vi "AssertValueByArrayPath.vi"(0 "VI Reference In":refnum<vi>, 1 "Test Label":string, 2 "delimiter (>>)":string=">>", 3 "Assert Only? (F)":bool, 5 "Control Path":string, 7 "Focus Item Path":string[](array[string]), 11 "Error In":errorcluster, 12 "Assert Interval(10 ms)":u32=10, 13 "Timeout(5 sec)":dbl=5.0) -> (4 "VI Reference Out":refnum<vi>, 6 "Asserted Value":string[](array[string]), 15 "Error Out":errorcluster)   [LabVIEW 2016, in "Drona.lvlib" / "AssertControlValue.lvlib" / "AssertTree.lvlib"]
doc: "Asserts if the focus item names given as a array of hierarchical path for multi-select tree controls are equal.\n\nHierarchical path represent their corresponding parents of an item from its origin. Use the delimiters '>>' between each hierarchy in the path.\n\nFor example to select the item 'Child3', give the hierarchical path as \"<b>Parent1</b>(top level parent in tree)<b>>>Child1</b>(children for parent1)<b>>>Child2</b>(children for child1)<b>>>Child3</b>(children for child2)\"\n\nThe input control name is given as a string , incase of path, use delimiters inbetween the path.\nThis VI gets the value of the control, untill the value is equal to the input value."
uses:
  AssertTree.lvlib
  Get/GetControlRef/GetControlRefByPath.vi
  <vilib>/Utility/error.llb/Error Cluster From Error Code.vi
  <vilib>/addons/_JKI Toolkits/Caraya/classes/Assert/Assert Equal Value_Variant.vi
  <vilib>/ErrorRing/Error Ring.xnode
  Get/GetControlRef/GetControlRef.lvlib
  <vilib>/addons/_JKI Toolkits/Caraya/classes/Assert/Assert.lvclass
  Drona.lvlib
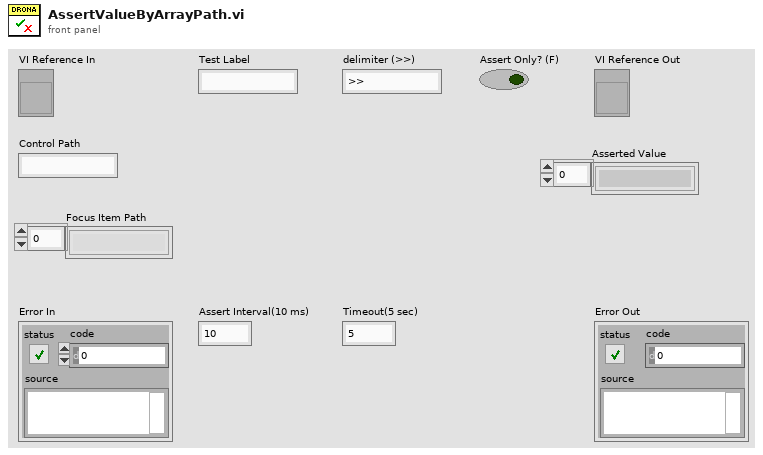
[diagram p1: front panel]
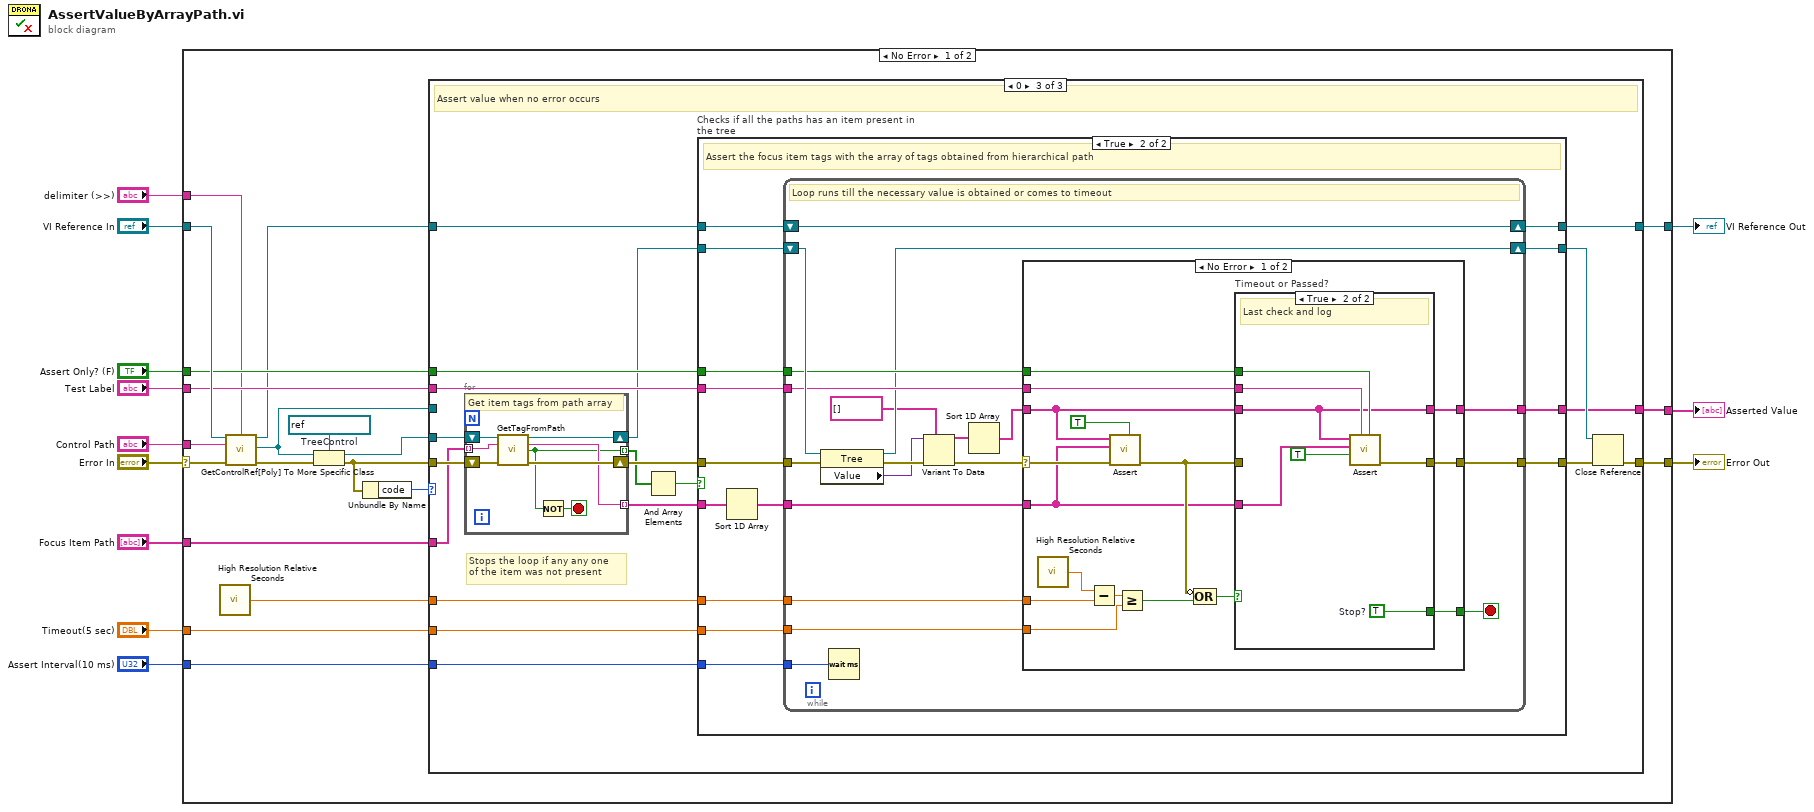
[diagram p0: block diagram]
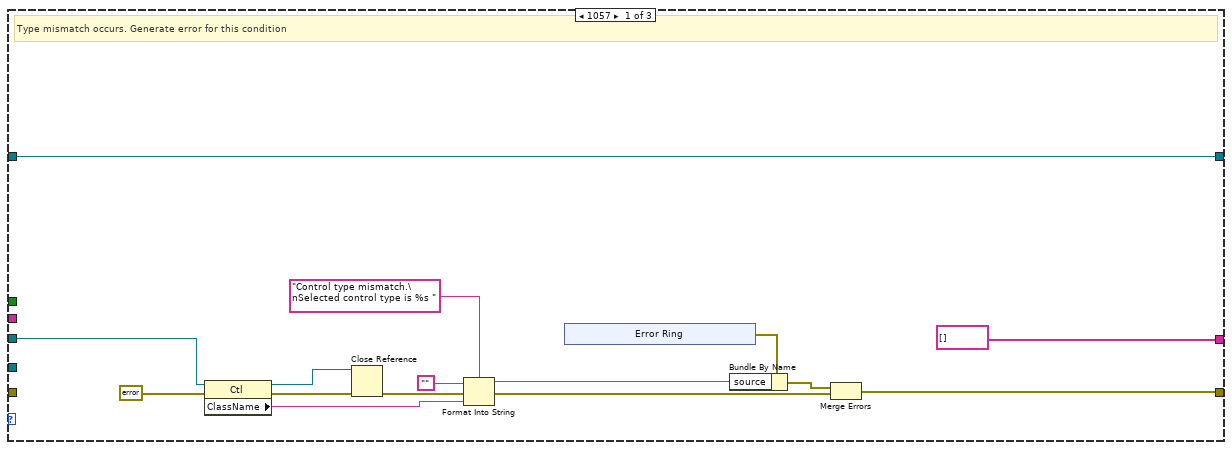
[diagram p2: hidden frame]
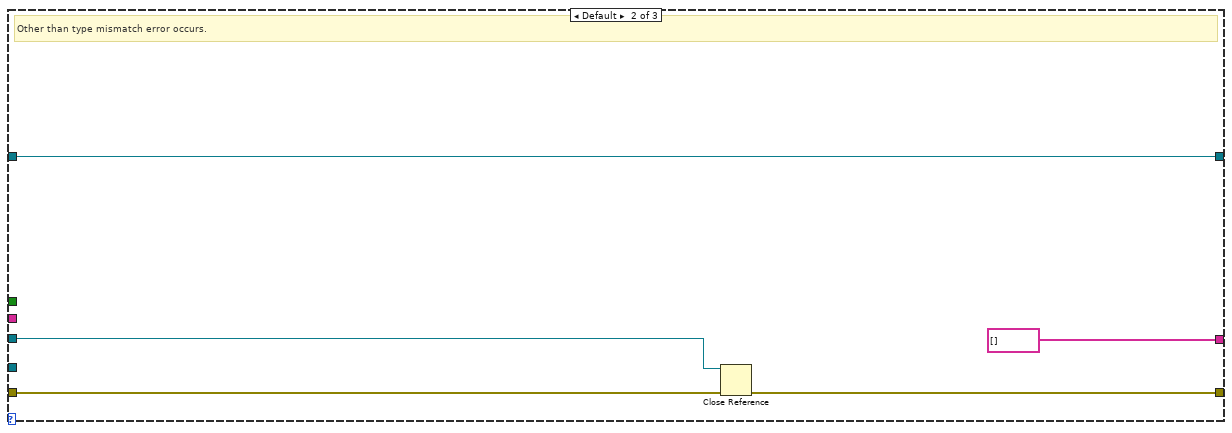
[diagram p3: hidden frame]
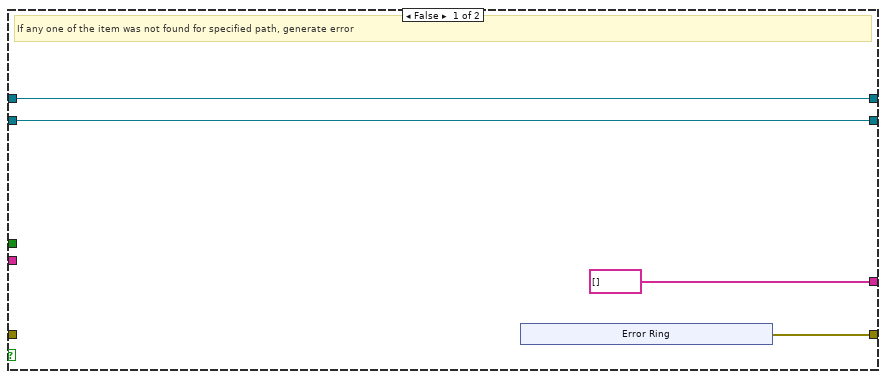
[diagram p4: hidden frame]
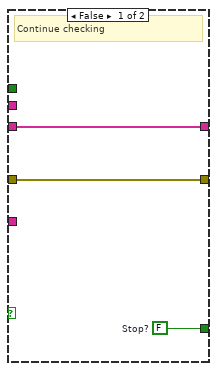
[diagram p5: hidden frame]
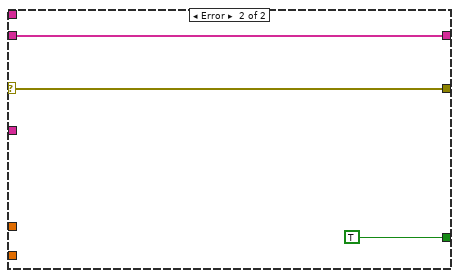
[diagram p6: hidden frame]
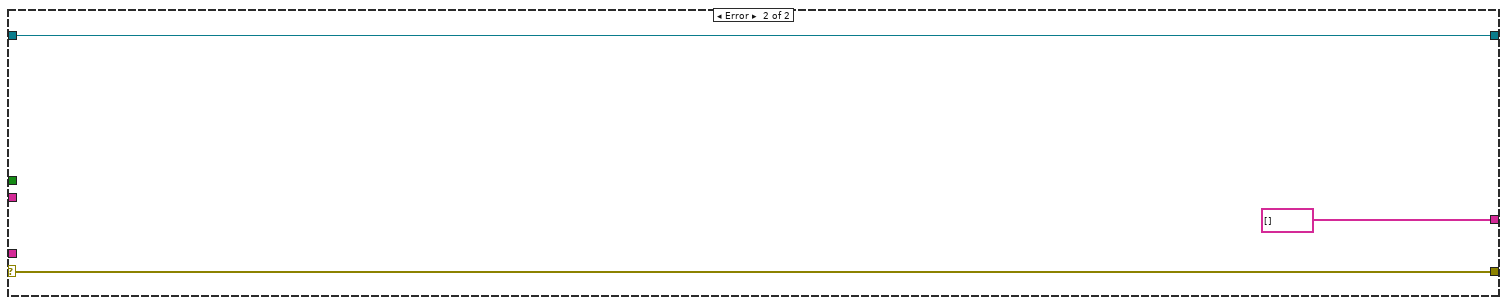
[diagram p7: hidden frame]
diagram:
  n1 = case shown="No Error" "Error In" {
    selector: "Error In" -> [w32 w158]
    tunnel: "Timeout(5 sec)" -> [w19 _]
    tunnel: [w17 w157] -> w11
    tunnel: "Focus Item Path" -> [w21 _]
    tunnel: [w15 w158] -> w10
    tunnel: "Assert Interval(10 ms)" -> [w18 _]
    tunnel: "Test Label" -> [w25 _]
    tunnel: "VI Reference In" -> [w31 w157]
    tunnel: "Control Path" -> [w13 _]
    tunnel: "delimiter (>>)" -> [w14 _]
    tunnel: "Assert Only? (F)" -> [w24 _]
    tunnel: [w16 string[] []] -> w1
    frame No Error {
      w29 = refnum<vi> refnum  # TreeControl
      n2 = call <vilib>:"High Resolution Relative Seconds.vi"() -> ("relative seconds"=w20:dbl)
      n3 = call-poly "GetControlRef[Poly].vi"("VI Reference In"=w31, "delimiter (>>)"=w14, "Control Path"=w13, "error In"=w32) -> ("VI Reference Out"=w23:refnum<vi>, "Ctl Refnum"=w26:refnum<vi>, "error out"=w30:errorcluster)  [unwired: 9 in]
      n4 = To More Specific Class(target class=w29, reference=w26, error in=w30) -> (specific class reference=w27:refnum<vi>, error out=w28:errorcluster)
      n5 = Unbundle By Name(w28) -> ("code"=w22:i32)
      n6 = case shown="0" w22 {
        tunnel: w19 -> [_ _ w76]
        tunnel: [w47 w57 w75] -> w17
        tunnel: w21 -> [_ _ w60]
        tunnel: w18 -> [_ _ w73]
        tunnel: w25 -> [_ _ w72]
        tunnel: w20 -> [_ _ w71]
        tunnel: w23 -> [w47 w57 w70]
        tunnel: [w35 w55 w69] -> w15
        tunnel: w24 -> [_ _ w67]
        tunnel: [string[] [] string[] [] w66] -> w16
        tunnel: w28 -> [_ w56 w65]
        tunnel: w27 -> [_ _ w64]
        tunnel: w26 -> [w34 w54 _]
        frame 1057 {
          # "Type mismatch occurs. Generate error for this condition"
          n7 = property class="Ctl"(reference=w34, error in=errorcluster {"status"=FALSE, "code"=0, "source"=""} ("error out")) -> (reference out=w36:refnum<vi>, error out=w46:errorcluster, "ClassName"=w43:string)
          n8 = Close Reference(reference=w36, error in (no error)=w46) -> (error out=w37:errorcluster)
          n9 = Format Into String(format string="Control type mismatch.\nSelected control type is %s ", initial string="", error in=w37, w43) -> (resulting string=w40:string, error out=w38:errorcluster)
          n10 = xnode "Error Ring"() -> ("error out"=w41:errorcluster)
          n11 = Bundle By Name(cluster=w41, "source"=w40) -> (w39:errorcluster)
          n12 = Merge Errors(w39, w38) -> (w35:errorcluster)
        }
        frame Default {
          # "Other than type mismatch error occurs."
          n13 = Close Reference(reference=w54, error in (no error)=w56) -> (error out=w55:errorcluster)
        }
        frame 0 {
          # "Stops the loop if any any one \nof the item was not present"
          # "Assert value when no error occurs"
          n14 = for {
            tunnel: [w78] -> w63 mode=indexing
            tunnel: [w77] -> w58 mode=indexing
            shift-right: [w82] -> w62
            shift-left: w65 -> [w83]
            shift-right: [w79] -> w61
            shift-left: w64 -> [w81]
            tunnel: w60 -> [w80] mode=indexing
            stop <- w84 stop-if-true
            # "Get item tags from path array"
            n15 = call "GetTagFromPath.vi"("Tree Ref In"=w81, "Hierarchical Path"=w80, "Error In"=w83) -> ("Tree Ref Out"=w79:refnum<vi>, "Item Tag"=w78:string, "Item Found?"=w77:bool, "Error Out"=w82:errorcluster)  [unwired: 9 in]
            n16 = Not(x=w77) -> (.not. x?=w84:bool)
          }
          n17 = And Array Elements(Boolean array=w58) -> (logical AND=w59:bool)
          n18 = case "Checks if all the paths has an item present in the tree" shown="True" w59 {
            tunnel: w76 -> [_ w107]
            tunnel: [w88 w106] -> w75
            tunnel: [w86 w105] -> w74
            tunnel: w73 -> [_ w104]
            tunnel: w72 -> [_ w103]
            tunnel: w71 -> [_ w102]
            tunnel: w70 -> [w88 w101]
            tunnel: [w87 w100] -> w68
            tunnel: w67 -> [_ w99]
            tunnel: [string[] [] w98] -> w66
            tunnel: w63 -> [_ w95]
            tunnel: w61 -> [w87 w96]
            tunnel: w62 -> [_ w97]
            frame False {
              # "If any one of the item was not found for specified path, generate error"
              n19 = xnode "Error Ring"() -> ("error out"=w86:errorcluster)
            }
            frame True {
              # "Assert the focus item tags with the array of tags obtained from hierarchical path"
              n20 = Sort 1D Array(array=w95) -> (sorted array=w94:string[])
              n21 = while {
                tunnel: w94 -> [w114]
                tunnel: w107 -> [w125]
                tunnel: w102 -> [w126]
                tunnel: w97 -> [w120]
                tunnel: [w123] -> w105
                tunnel: w104 -> [w121]
                tunnel: w103 -> [w117]
                shift-right: [w118] -> w106
                shift-left: w101 -> [w118]
                shift-right: [w111] -> w100
                shift-left: w96 -> [w119]
                tunnel: w99 -> [w116]
                tunnel: [w115] -> w98
                stop <- w124 stop-if-true
                # "Loop runs till the necessary value is obtained or comes to timeout"
                n22 = property on="Property Node" class="Tree"(reference=w119, error in=w120) -> (reference out=w111:refnum<vi>, error out=w122:errorcluster, "Value"=w112:variant)
                n23 = Wait (ms)(milliseconds to wait=w121) -> ()  [unwired: 1 out]
                n24 = Variant To Data(error in=w122, type=string[] [], Variant=w112) -> (data=w109:string[], error out=w113:errorcluster)
                n25 = Sort 1D Array(array=w109) -> (sorted array=w108:string[])
                n26 = case shown="No Error" w113 {
                  selector: w113 -> [w138 w155]
                  tunnel: w126 -> [w142 _]
                  tunnel: w125 -> [w139 _]
                  tunnel: [w129 TRUE] -> w124
                  tunnel: [w130 w155] -> w123
                  tunnel: w114 -> [w131 _]
                  tunnel: w108 -> [w132 w153]
                  tunnel: w117 -> [w137 _]
                  tunnel: w116 -> [w128 _]
                  tunnel: [w127 w153] -> w115
                  frame No Error {
                    n27 = call <vilib>:"High Resolution Relative Seconds.vi"() -> ("relative seconds"=w141:dbl)
                    n28 = Subtract(x=w141, y=w142) -> (x-y=w140:dbl)
                    n29 = call-poly <vilib>:"Assert.vi"("Assert Only? (F)"=TRUE, "error in (no error)"=w138, "Y"=w131, "X"=w132) -> ("error out"=w135:errorcluster)  [unwired: 6 in, 1 out]
                    n30 = Greater Or Equal?(x=w140, y=w139) -> (x >= y?=w136:bool)
                    n31 = Compound Arithmetic op=OR(invert w135, w136) -> (w134:bool)
                    n32 = case "Timeout or Passed?" shown="True" w134 {
                      tunnel: w135 -> [w145 _]
                      tunnel: w131 -> [_ w148]
                      tunnel: w132 -> [w143 w147]
                      tunnel: w137 -> [_ w152]
                      tunnel: [w145 w151] -> w130
                      tunnel: [w144 w150] -> w129
                      tunnel: w128 -> [_ w149]
                      tunnel: [w143 w147] -> w127
                      frame False {
                        w144 = FALSE  # Stop?
                        # "Continue checking"
                      }
                      frame True {
                        w150 = TRUE  # Stop?
                        # "Last check and log"
                        n33 = call-poly <vilib>:"Assert.vi"("Assert Only? (F)"=w149, "Label"=w152, "Register with caller test (F)"=TRUE, "Y"=w148, "X"=w147) -> ("error out"=w151:errorcluster)  [unwired: 5 in, 1 out]
                      }
                    }
                  }
                  frame Error {
                  }
                }
              }
            }
          }
          n34 = Close Reference(reference=w68, error in (no error)=w74) -> (error out=w69:errorcluster)
        }
      }
    }
    frame Error {
    }
  }
  "Error Out" <- w10
  "VI Reference Out" <- w11
  "Asserted Value" <- w1
